vi "uActor_SendNestedStopped.vi"(8 "error in (no error)":errorcluster, 11 "uActor Last State":refnum<class "uActor.lvclass">) -> (0 "error out":errorcluster, 3 "uActor out":refnum<class "uActor.lvclass">)   [LabVIEW 2023, in "uLib.lvlib" / "uActor.lvclass"]
doc: "Wrap the last actor state and the last error state in a message and send to the caller.\nThis VI executes regardless of the error state and does not return an error if the caller actor transport is invalid."
uses:
  uActor.lvclass
  uActor.lvclass/uActor.ctl
  uData/uData/uData.lvclass
  uData/uData/uData.lvclass/uData.ctl
  uMsg/uMsg/uMsg.lvclass/uMsg.ctl
  uTransport/uTransport_uActor/uTransport_uActor.lvclass/uTransport_uActor.ctl
  uTransport/uTransport_uActor/uTransport_uActor_SendMsg.vi
  uMsg/uMsg/uMsg Update Timestamp.vi
  uData/uData/Condition Tag Name.vi
  uData/uData/Blank Key Reserved String.vi
  uTransport/uTransport/uTransport.lvclass
  uMsg/uMsg/uMsg.lvclass
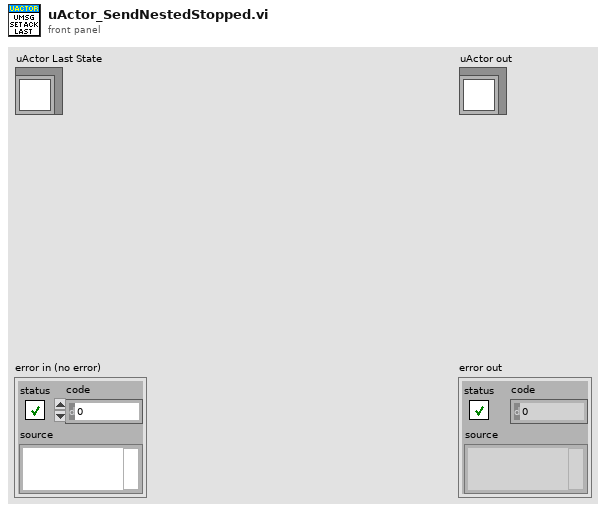
[diagram p1: front panel]
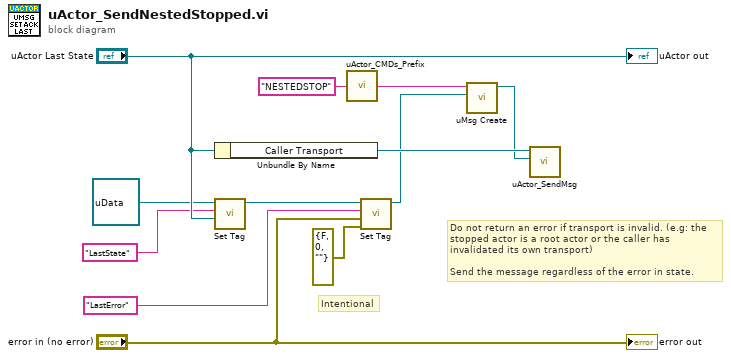
[diagram p0: block diagram]
diagram:
  # "Intentional"
  # "Do not return an error if transport is invalid. (e.g: the stopped actor is a root actor or the caller has invalidated its own transport)\n\nSend the message regardless of the error in state."
  n1 = Unbundle By Name("uActor Last State") -> ("Caller Transport"=w9:refnum<class "uTransport_uActor.lvclass">)
  n2 = call "Set Tag.vi"("Variant"="uActor Last State", "tag (case insensitive)"="LastState" ("uMsg Tag"), "uData in"=refnum<class "uData.lvclass"> refnum) -> ("uData out"=w7:refnum<class "uData.lvclass">)  [unwired: 6 in, 2 out]
  n3 = call "uActor_CMDs_Prefix.vi"("uActor CMD"="NESTEDSTOP") -> ("Reserved CMD"=w5:string)
  n4 = call "Set Tag.vi"("error in (no error)"=errorcluster {"status"=FALSE, "code"=0, "source"=""}, "Variant"="error in (no error)", "tag (case insensitive)"="LastError" ("uMsg Tag"), "uData in"=w7) -> ("uData out"=w3:refnum<class "uData.lvclass">)  [unwired: 5 in, 2 out]
  n5 = call "uMsg Create.vi"("Payload"=w3, "CMD"=w5) -> ("uMsg out"=w4:refnum<class "uMsg.lvclass">)  [unwired: 8 in, 1 out]
  n6 = call "uActor_SendMsg.vi"("Msg"=w4, "uActor Transport"=w9) -> ()  [unwired: 9 in, 1 out]
  "error out" <- "error in (no error)"
  "uActor out" <- "uActor Last State"
